vi "Auto_Inspection Station MainS4.vi"(8 "站別":refnum<vi>, 9 "站別":i32, 10 "ActRef":refnum<vi>, 11 "Station Action.lvclass":refnum<class "Station Action.lvclass">) -> ()   [LabVIEW 2019]
uses:
  Station Class/Station Action.lvclass
  Ctrl/Station Action.ctl
  Ctrl/Auto Inspection Data Name.ctl
  FlowCtrl Class/BarcodeScan/Ctl/Board Scan IO.ctl
  FlowCtrl Class/Ctrl/Auto Inspection_IN Name2.ctl
  Ctrl/ModbusCmd.ctl
  Ctrl/S2 Station IO.ctl
  FlowCtrl Class/Laser Detect/Ctl/S11 Station IO.ctl
  Function/Main UI/Glb/Main_UI Gb.vi
  Global/Process Global.vi
  Ctrl/Auto Inspection Main UI Ref.ctl
  LLB/Commonly VI.lvlib
  Ctrl/Auto Inspection Station Name2.ctl
  LLB/Commonly VI/Main Glb.vi
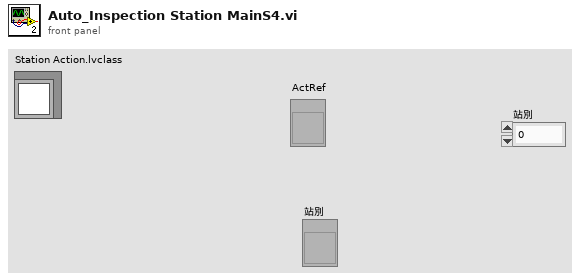
[diagram p1: front panel]
types:
  T1 = typedef "Station Action.ctl" = enum16{"Wait Item In", "Dectect Action", "ImformOut"}
  T2 = cluster{"AutoRunFlg":refnum<vi>, "Action Finish Flg":refnum<vi>, "Remaining Action":refnum<vi>, "Btn_AutoRun":refnum<vi>, "Manual Flg":refnum<vi>, "Sub Process Error":refnum<vi>}
  T3 = typedef "Auto Inspection Data Name.ctl" = enum16{"LocalRun", "ItemSN(TimeCode)", "CurrentAction", "Error", "Data", "OKNG", "電壓值", "電壓值判斷", "電流值", "電流值判斷", "Laser1 Data", "Laser2 Data", "Laser OKNG", "StationNO"}
  T4 = cluster{"starting address":u16, "number of inputs":u16, "Sat Coils":bool[], "Holding Registers":u16[]}
  T5 = typedef "ModbusCmd.ctl" = enum16{"Connect", "Disconnect", "Init", "Fetch Basic Objects", "Fetch Input Refisters", "Fetch Discrete Inputs", "Set Coils", "Set Holding Registers", "Write Single Holding", "Exit"}
  T6 = typedef "Auto Inspection_IN Name2.ctl" = enum16{"S0 Station", "S1 Barcode ", "S2 Tool Format", "S3 Tool Prpgram", "S4 Tool Sacn", "S11 Laser Detect", "S8 Vision AI"}
  T7 = typedef "Board Scan IO.ctl" = enum16{"S1 Barcode Scan", "回給PLC完成讀取訊號", "S1 載盤條碼比對NG", "S1PLC 條碼可讀取訊號", "S1備用_04", "S1備用_05", "S1備用_06", "S1備用_07", "S1備用_08", "S1 發送條碼完成"}
  T8 = typedef "S2 Station IO.ctl" = enum16{"S2站PC動作中_20", "電流量測完成產品OK_21", "電流量測完成產品NG_22", "S2站Format 執行_23", "S2 Format OK_24", "S2 Format NG_25", "S2站燒入執行_26", "S2站燒入OK_27", "S2站燒入NG_28", "S2站動作完成_29", "S3 PC動作中_30", "S3 Format 此站執行_31", "S3 Format OK_32", "S3 Format NG_33", "S3 燒入程式 此站執行_34", "S3 燒入程式 OK_35", "S3 燒入程式 NG_36", "S3 備用_37", "S3 備用_38", "S3 動作完成_39", "S4 PC動作中_40", "S4 量測完成 產品正常_41", "S4 量測完成 產品NG_42", "S4 Format 此站執行_43", "S4 Format OK_44", "S4 Format NG_45", "S4 燒入 此站不執行_46", "S4 燒入程式 OK_47", "S4 燒入程式 NG_48", "S4 藍芽Scan OK_49", "S4 藍芽Scan NG_50", "S4 動作完成_51", "給PLC要量電流訊號", "給PLC要量電壓訊號"}
  T9 = typedef "S11 Station IO.ctl" = enum16{"S11雷射測量動作中", "S11雷射測點1完成", "S11雷射測點2完成", "S11雷測測量OK", "S11雷測測量NG", "S11雷測測量重測", "S11備用_6", "S11備用_7", "S11備用_8", "S11雷射測高完成"}
  T10 = typedef "Auto Inspection Station Name2.ctl" = enum16{"S1Barcode", "S2Measure", "S3Measure", "S4Measure", "S5Measure", "S11_LaserCheck", "S8_Vision AI"}
  T11 = typedef "Auto Inspection Main UI Ref.ctl" = cluster{"LineScan arrive":refnum<vi>, "LineScanfinish":refnum<vi>, "AI arrive":refnum<vi>, "AI finish":refnum<vi>, "NG Pick arrive":refnum<vi>, "NG Pick finish":refnum<vi>}
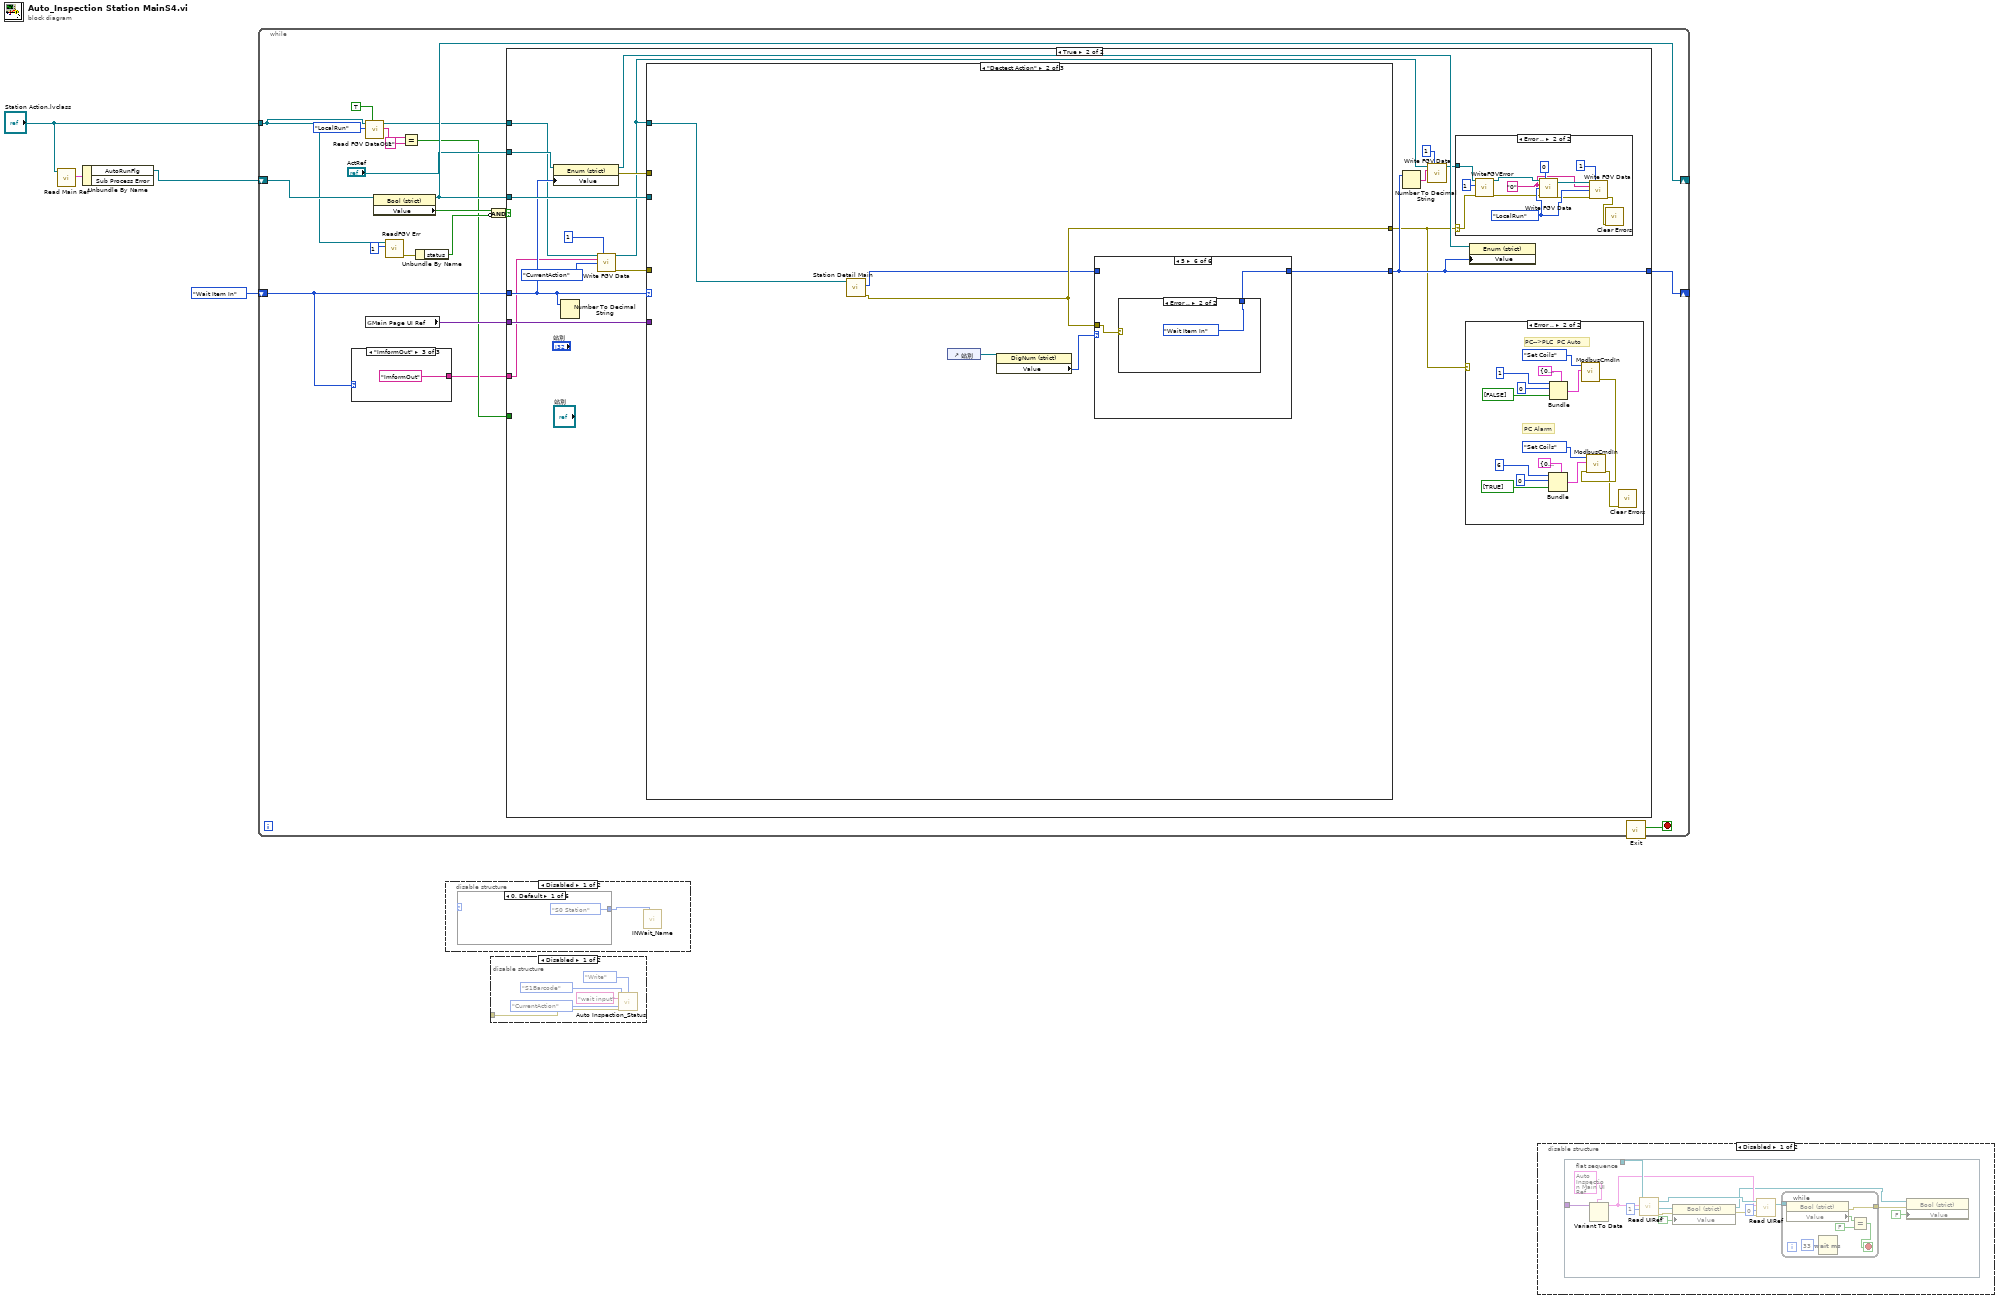
[diagram p0: block diagram]
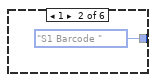
[diagram p2: hidden frame]
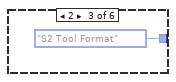
[diagram p3: hidden frame]
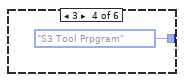
[diagram p4: hidden frame]
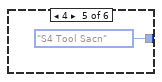
[diagram p5: hidden frame]
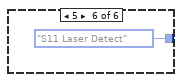
[diagram p6: hidden frame]
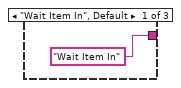
[diagram p10: hidden frame]
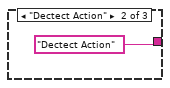
[diagram p11: hidden frame]
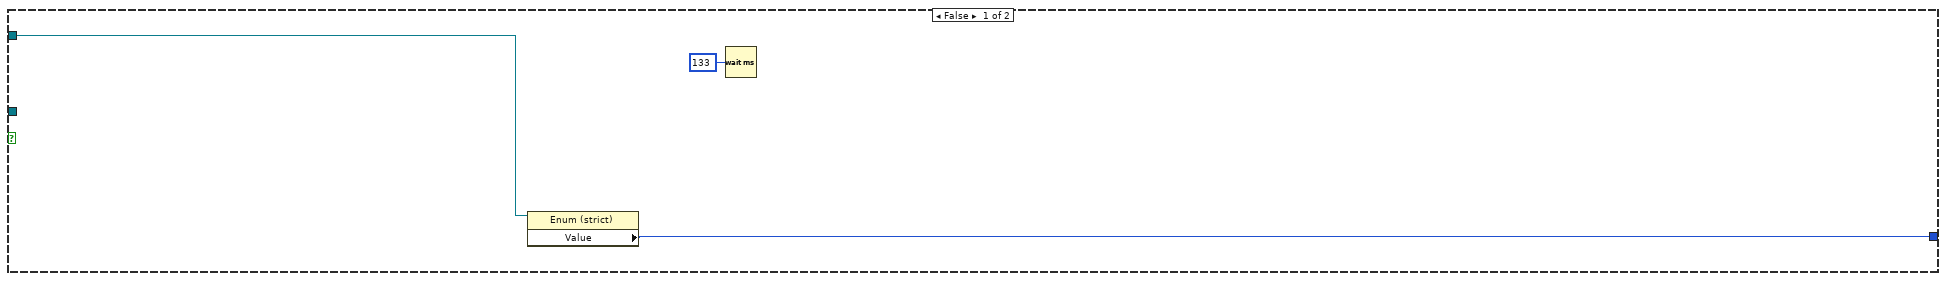
[diagram p12: hidden frame]
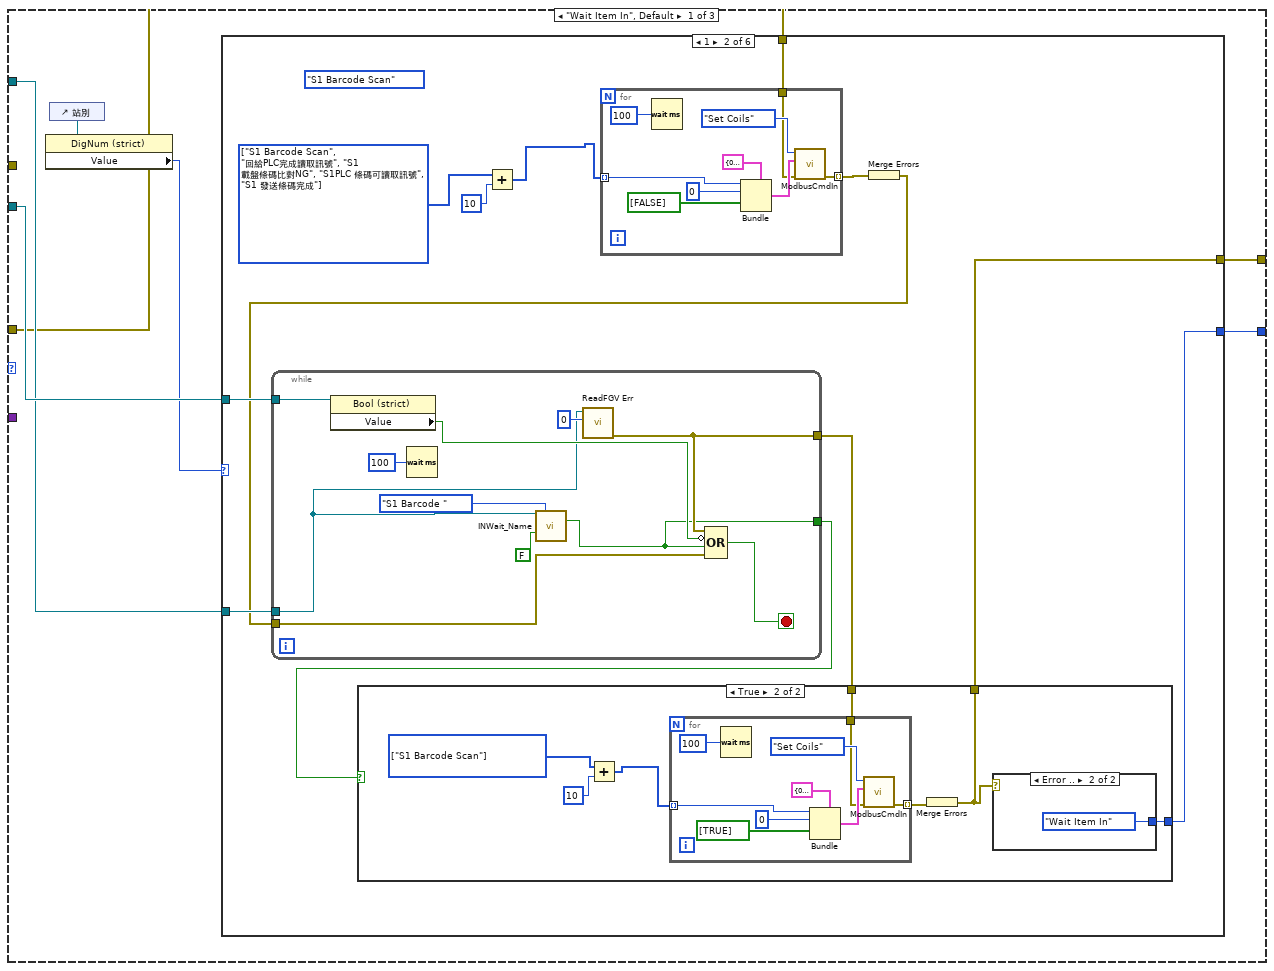
[diagram p15: hidden frame]
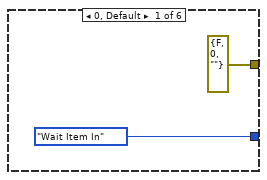
[diagram p16: hidden frame]
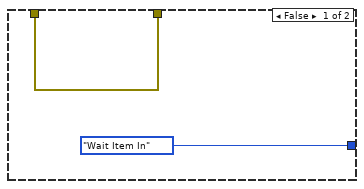
[diagram p17: hidden frame]
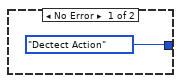
[diagram p18: hidden frame]
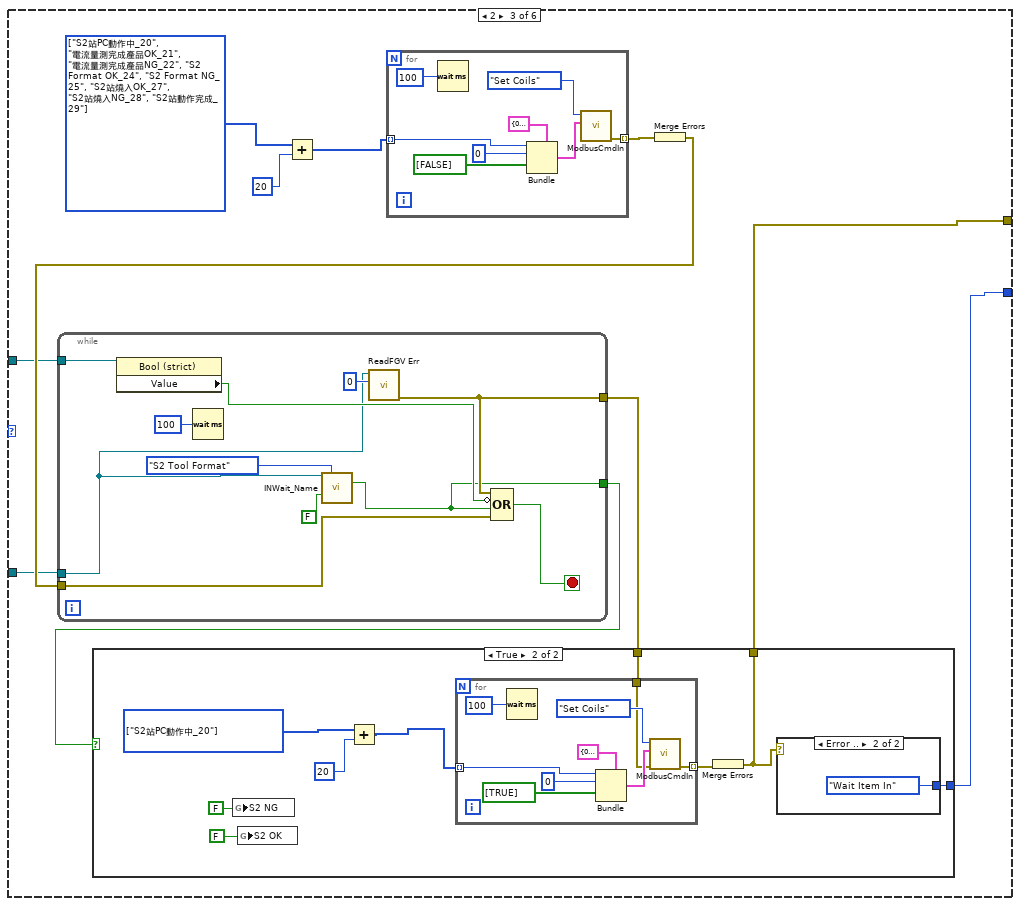
[diagram p19: hidden frame]
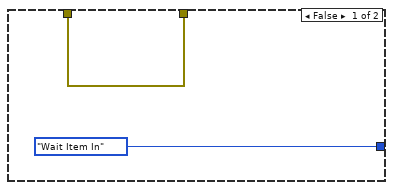
[diagram p20: hidden frame]
diagram:
  n1 = call-dynamic "Read Main Ref.vi"("Main Process Class in"="Station Action.lvclass") -> ("Main Ref"=w3:T2)  [unwired: 8 in, 2 out]
  n2 = Unbundle By Name(w3) -> ("AutoRunFlg"=w1:refnum<vi>)  [unwired: 1 out]
  n3 = while {
    shift-right: [w20] -> _
    shift-left: Station_Action."Wait Item In" -> [w6]
    tunnel: "Station Action.lvclass" -> [w8]
    shift-right: [w18] -> _
    shift-left: w1 -> [w23]
    stop <- w19 stop-if-true
    n4 = case shown="\"ImformOut\"" w6 {
      tunnel: ["Wait Item In" "Dectect Action" "ImformOut"] -> w5
      frame "Wait Item In", Default {
      }
      frame "Dectect Action" {
      }
      frame "ImformOut" {
      }
    }
    n5 = call-dynamic "Read FGV DataOut.vi"("TSt/FConveyor"=TRUE, "Data"=Auto_Inspection_Data_Name."LocalRun", "Station Action in"=w8) -> ("DataOut"=w11:string, "Station Action out"=w14:refnum<class "Station Action.lvclass">)  [unwired: 6 in, 1 out]
    n6 = global read "Main_UI Gb.vi" "Main Page UI Ref"() -> (w21:variant)
    n7 = property class="Bool (strict)"(reference=w23) -> (reference out=w18:refnum<vi>, "Value"=w24:bool)  [unwired: 1 in, 1 out]
    n8 = call-dynamic "ReadFGV Err.vi"("0Cv/1ST"=1, "Station Action in"=w8) -> ("error out"=w16:errorcluster)  [unwired: 8 in, 1 out]
    n9 = Equal?(x=w11, y="1") -> (x = y?=w7:bool)
    n10 = Unbundle By Name(w16) -> ("status"=w15:bool)
    n11 = Compound Arithmetic op=AND(w24, invert w15) -> (w22:bool)
    n12 = case shown="True" w22 {
      tunnel: w18 -> [_ w46]
      tunnel: w6 -> [_ w39]
      tunnel: w21 -> [_ w47]
      tunnel: w14 -> [_ w32]
      tunnel: [w29 w36] -> w20
      tunnel: "ActRef" -> [w30 w45]
      tunnel: w7 -> [_ _]
      tunnel: w5 -> [_ w31]
      frame False {
        n13 = property class="Enum (strict)"(reference=w30) -> ("Value"=w29:T1)  [unwired: 1 in, 2 out]
        n14 = Wait (ms)(milliseconds to wait=u32 133) -> ()  [unwired: 1 out]
      }
      frame True {
        n15 = property class="Enum (strict)"(reference=w45, "Value"=w39) -> (reference out=w44:refnum<vi>, error out=w43:errorcluster)  [unwired: 1 in]
        n16 = Number To Decimal String(number=w39) -> ()  [unwired: 1 in, 1 out]
        n17 = call-dynamic "Write FGV Data.vi"("Station Action in"=w32, "0Cv/1St"=1, "DataIn"=w31, "Data"=Auto_Inspection_Data_Name."CurrentAction") -> ("Station Action out"=w35:refnum<class "Station Action.lvclass">, "error out"=w40:errorcluster)  [unwired: 10 in]
        n18 = case shown="\"Dectect Action\"" w39 {
          tunnel: w47 -> [_ _ _]
          tunnel: w35 -> [w79 w350 w378]
          tunnel: w46 -> [w80 _ w377]
          tunnel: [w75 w348 w373] -> w36
          tunnel: w43 -> [_ _ _]
          tunnel: [w78 w349 w374] -> w33
          tunnel: w40 -> [w74 _ w376]
          frame "Wait Item In", Default {
            n19 = control-ref of="站別"() -> (w77:refnum<vi>)
            n20 = property class="DigNum (strict)"(reference=w77) -> ("Value"=w76:i32)  [unwired: 1 in, 2 out]
            n21 = case shown="1" w76 {
              tunnel: w80 -> [_ w94 w139 w193 w245 w296]
              tunnel: w79 -> [_ w93 w140 w192 w244 w298]
              tunnel: [errorcluster {"status"=FALSE, "code"=0, "source"=""} ("error IO") w92 w142 w195 w241 w297] -> w78
              tunnel: w74 -> [_ w91 _ w188 w246 w299]
              tunnel: [Station_Action."Wait Item In" w87 w141 w194 w243 w294] -> w75
              frame 0, Default {
              }
              frame 1 {
                (unwired) Board_Scan_IO."S1 Barcode Scan" ("Enum")
                w85 = T7[] [enum."S1 Barcode Scan", enum."回給PLC完成讀取訊號", enum."S1 載盤條碼比對NG", enum."S1PLC 條碼可讀取訊號", enum."S1 發送條碼完成"] items=["S1 Barcode Scan", "回給PLC完成讀取訊號", "S1 載盤條碼比對NG", "S1PLC 條碼可讀取訊號", "S1備用_04", "S1備用_05", "S1備用_06", "S1備用_07", "S1備用_08", "S1 發送條碼完成"]
                n22 = Add(x=w85, y=10) -> (x+y=w84:i32[])
                n23 = for {
                  tunnel: [w128] -> w90 mode=indexing
                  tunnel: w84 -> [w127] mode=indexing
                  tunnel: w91 -> [w126]
                  n24 = Wait (ms)(milliseconds to wait=100) -> ()  [unwired: 1 out]
                  n25 = Bundle(cluster=T4 {"starting address"=0, "number of inputs"=0, "Sat Coils"=[], "Holding Registers"=[]} ("data"), "starting address"=w127, "number of inputs"=u16 0, "Sat Coils"=bool[] [FALSE]) -> (w131:T4)  [unwired: 1 in]
                  n26 = call "ModbusCmdIn.vi"("error in (no error)"=w126, "data"=w131, "Enum"=ModbusCmd."Set Coils") -> ("error out"=w128:errorcluster)  [unwired: 8 in]
                }
                n27 = Merge Errors(w90) -> (w89:errorcluster)
                n28 = while {
                  tunnel: w94 -> [w125]
                  tunnel: w93 -> [w119]
                  tunnel: [w120] -> w88
                  tunnel: w89 -> [w117]
                  tunnel: [w116] -> w83
                  stop <- w124 stop-if-true
                  n29 = property class="Bool (strict)"(reference=w125) -> ("Value"=w122:bool)  [unwired: 1 in, 2 out]
                  n30 = Wait (ms)(milliseconds to wait=u32 100) -> ()  [unwired: 1 out]
                  n31 = call "INWait_Name.vi"("FlowCtrl in"=w119, "Input2"=Auto_Inspection_IN_Name2."S1 Barcode ", "Wait?"=FALSE) -> ("StatusOut"=w116:bool)  [unwired: 9 in, 3 out]
                  n32 = call-dynamic "ReadFGV Err.vi"("0Cv/1ST"=0, "Station Action in"=w119) -> ("error out"=w120:errorcluster)  [unwired: 8 in, 1 out]
                  n33 = Compound Arithmetic op=OR(w120, invert w122, w116, w117) -> (w124:bool)
                }
                n34 = case shown="True" w83 {
                  tunnel: [w96 w97] -> w92
                  tunnel: w88 -> [w96 w103]
                  tunnel: [Station_Action."Wait Item In" w100] -> w87
                  frame False {
                  }
                  frame True {
                    w99 = T7[] [enum."S1 Barcode Scan"] items=["S1 Barcode Scan", "回給PLC完成讀取訊號", "S1 載盤條碼比對NG", "S1PLC 條碼可讀取訊號", "S1備用_04", "S1備用_05", "S1備用_06", "S1備用_07", "S1備用_08", "S1 發送條碼完成"]
                    n35 = Add(x=w99, y=10) -> (x+y=w102:i32[])
                    n36 = for {
                      tunnel: [w108] -> w101 mode=indexing
                      tunnel: w102 -> [w107] mode=indexing
                      tunnel: w103 -> [w106]
                      n37 = Wait (ms)(milliseconds to wait=100) -> ()  [unwired: 1 out]
                      n38 = Bundle(cluster=T4 {"starting address"=0, "number of inputs"=0, "Sat Coils"=[], "Holding Registers"=[]} ("data"), "starting address"=w107, "number of inputs"=u16 0, "Sat Coils"=bool[] [TRUE]) -> (w111:T4)  [unwired: 1 in]
                      n39 = call "ModbusCmdIn.vi"("error in (no error)"=w106, "data"=w111, "Enum"=ModbusCmd."Set Coils") -> ("error out"=w108:errorcluster)  [unwired: 8 in]
                    }
                    n40 = Merge Errors(w101) -> (w97:errorcluster)
                    n41 = case shown="Error .." w97 {
                      tunnel: [Station_Action."Dectect Action" Station_Action."Wait Item In"] -> w100
                      frame No Error {
                      }
                      frame Error {
                      }
                    }
                  }
                }
              }
              frame 2 {
                w137 = T8[] [enum."S2站PC動作中_20", enum."電流量測完成產品OK_21", enum."電流量測完成產品NG_22", enum."S2 Format OK_24", enum."S2 Format NG_25", enum."S2站燒入OK_27", enum."S2站燒入NG_28", enum."S2站動作完成_29"] items=["S2站PC動作中_20", "電流量測完成產品OK_21", "電流量測完成產品NG_22", "S2站Format 執行_23", "S2 Format OK_24", "S2 Format NG_25", "S2站燒入執行_26", "S2站燒入OK_27", "S2站燒入NG_28", "S2站動作完成_29", "S3 PC動作中_30", "S3 Format 此站執行_31", "S3 Format OK_32", "S3 Format NG_33", "S3 燒入程式 此站執行_34", "S3 燒入程式 OK_35", "S3 燒入程式 NG_36", "S3 備用_37", "S3 備用_38", "S3 動作完成_39", "S4 PC動作中_40", "S4 量測完成 產品正常_41", "S4 量測完成 產品NG_42", "S4 Format 此站執行_43", "S4 Format OK_44", "S4 Format NG_45", "S4 燒入 此站不執行_46", "S4 燒入程式 OK_47", "S4 燒入程式 NG_48", "S4 藍芽Scan OK_49", "S4 藍芽Scan NG_50", "S4 動作完成_51", "給PLC要量電流訊號", "給PLC要量電壓訊號"]
                n42 = Add(x=w137, y=20) -> (x+y=w136:i32[])
                n43 = for {
                  tunnel: [w180] -> w143 mode=indexing
                  tunnel: w136 -> [w179] mode=indexing
                  n44 = Wait (ms)(milliseconds to wait=100) -> ()  [unwired: 1 out]
                  n45 = Bundle(cluster=T4 {"starting address"=0, "number of inputs"=0, "Sat Coils"=[], "Holding Registers"=[]} ("data"), "starting address"=w179, "number of inputs"=u16 0, "Sat Coils"=bool[] [FALSE]) -> (w183:T4)  [unwired: 1 in]
                  n46 = call "ModbusCmdIn.vi"("data"=w183, "Enum"=ModbusCmd."Set Coils") -> ("error out"=w180:errorcluster)  [unwired: 9 in]
                }
                n47 = Merge Errors(w143) -> (w144:errorcluster)
                n48 = while {
                  tunnel: w140 -> [w173]
                  tunnel: [w174] -> w145
                  tunnel: w144 -> [w171]
                  tunnel: [w170] -> w135
                  tunnel: w139 -> [w168]
                  stop <- w178 stop-if-true
                  n49 = property class="Bool (strict)"(reference=w168) -> ("Value"=w176:bool)  [unwired: 1 in, 2 out]
                  n50 = Wait (ms)(milliseconds to wait=u32 100) -> ()  [unwired: 1 out]
                  n51 = call "INWait_Name.vi"("FlowCtrl in"=w173, "Input2"=Auto_Inspection_IN_Name2."S2 Tool Format", "Wait?"=FALSE) -> ("StatusOut"=w170:bool)  [unwired: 9 in, 3 out]
                  n52 = call-dynamic "ReadFGV Err.vi"("0Cv/1ST"=0, "Station Action in"=w173) -> ("error out"=w174:errorcluster)  [unwired: 8 in, 1 out]
                  n53 = Compound Arithmetic op=OR(w174, invert w176, w170, w171) -> (w178:bool)
                }
                n54 = case shown="True" w135 {
                  tunnel: w145 -> [w147 w155]
                  tunnel: [w147 w150] -> w142
                  tunnel: [Station_Action."Wait Item In" w154] -> w141
                  frame False {
                  }
                  frame True {
                    w153 = T8[] [enum."S2站PC動作中_20"] items=["S2站PC動作中_20", "電流量測完成產品OK_21", "電流量測完成產品NG_22", "S2站Format 執行_23", "S2 Format OK_24", "S2 Format NG_25", "S2站燒入執行_26", "S2站燒入OK_27", "S2站燒入NG_28", "S2站動作完成_29", "S3 PC動作中_30", "S3 Format 此站執行_31", "S3 Format OK_32", "S3 Format NG_33", "S3 燒入程式 此站執行_34", "S3 燒入程式 OK_35", "S3 燒入程式 NG_36", "S3 備用_37", "S3 備用_38", "S3 動作完成_39", "S4 PC動作中_40", "S4 量測完成 產品正常_41", "S4 量測完成 產品NG_42", "S4 Format 此站執行_43", "S4 Format OK_44", "S4 Format NG_45", "S4 燒入 此站不執行_46", "S4 燒入程式 OK_47", "S4 燒入程式 NG_48", "S4 藍芽Scan OK_49", "S4 藍芽Scan NG_50", "S4 動作完成_51", "給PLC要量電流訊號", "給PLC要量電壓訊號"]
                    n55 = global write "Process Global.vi" "S2 NG"(FALSE) -> ()
                    n56 = global write "Process Global.vi" "S2 OK"(FALSE) -> ()
                    n57 = Add(x=w153, y=20) -> (x+y=w151:i32[])
                    n58 = for {
                      tunnel: [w161] -> w156 mode=indexing
                      tunnel: w151 -> [w160] mode=indexing
                      tunnel: w155 -> [w159]
                      n59 = Wait (ms)(milliseconds to wait=100) -> ()  [unwired: 1 out]
                      n60 = Bundle(cluster=T4 {"starting address"=0, "number of inputs"=0, "Sat Coils"=[], "Holding Registers"=[]} ("data"), "starting address"=w160, "number of inputs"=u16 0, "Sat Coils"=bool[] [TRUE]) -> (w164:T4)  [unwired: 1 in]
                      n61 = call "ModbusCmdIn.vi"("error in (no error)"=w159, "data"=w164, "Enum"=ModbusCmd."Set Coils") -> ("error out"=w161:errorcluster)  [unwired: 8 in]
                    }
                    n62 = Merge Errors(w156) -> (w150:errorcluster)
                    n63 = case shown="Error .." w150 {
                      tunnel: [Station_Action."Dectect Action" Station_Action."Wait Item In"] -> w154
                      frame No Error {
                      }
                      frame Error {
                      }
                    }
                  }
                }
              }
              frame 3 {
                w191 = T8[] [enum."S3 PC動作中_30", enum."S3 Format OK_32", enum."S3 Format NG_33", enum."S3 燒入程式 OK_35", enum."S3 燒入程式 NG_36", enum."S3 動作完成_39"] items=["S2站PC動作中_20", "電流量測完成產品OK_21", "電流量測完成產品NG_22", "S2站Format 執行_23", "S2 Format OK_24", "S2 Format NG_25", "S2站燒入執行_26", "S2站燒入OK_27", "S2站燒入NG_28", "S2站動作完成_29", "S3 PC動作中_30", "S3 Format 此站執行_31", "S3 Format OK_32", "S3 Format NG_33", "S3 燒入程式 此站執行_34", "S3 燒入程式 OK_35", "S3 燒入程式 NG_36", "S3 備用_37", "S3 備用_38", "S3 動作完成_39", "S4 PC動作中_40", "S4 量測完成 產品正常_41", "S4 量測完成 產品NG_42", "S4 Format 此站執行_43", "S4 Format OK_44", "S4 Format NG_45", "S4 燒入 此站不執行_46", "S4 燒入程式 OK_47", "S4 燒入程式 NG_48", "S4 藍芽Scan OK_49", "S4 藍芽Scan NG_50", "S4 動作完成_51", "給PLC要量電流訊號", "給PLC要量電壓訊號"]
                n64 = Add(x=w191, y=20) -> (x+y=w189:i32[])
                n65 = for {
                  tunnel: [w233] -> w196 mode=indexing
                  tunnel: w189 -> [w232] mode=indexing
                  tunnel: w188 -> [w231]
                  n66 = Wait (ms)(milliseconds to wait=100) -> ()  [unwired: 1 out]
                  n67 = Bundle(cluster=T4 {"starting address"=0, "number of inputs"=0, "Sat Coils"=[], "Holding Registers"=[]} ("data"), "starting address"=w232, "number of inputs"=u16 0, "Sat Coils"=bool[] [FALSE]) -> (w236:T4)  [unwired: 1 in]
                  n68 = call "ModbusCmdIn.vi"("error in (no error)"=w231, "data"=w236, "Enum"=ModbusCmd."Set Coils") -> ("error out"=w233:errorcluster)  [unwired: 8 in]
                }
                n69 = Merge Errors(w196) -> (w197:errorcluster)
                n70 = while {
                  tunnel: w193 -> [w230]
                  tunnel: w192 -> [w224]
                  tunnel: [w225] -> w198
                  tunnel: w197 -> [w222]
                  tunnel: [w221] -> w187
                  stop <- w229 stop-if-true
                  n71 = property class="Bool (strict)"(reference=w230) -> ("Value"=w227:bool)  [unwired: 1 in, 2 out]
                  n72 = Wait (ms)(milliseconds to wait=u32 100) -> ()  [unwired: 1 out]
                  n73 = call "INWait_Name.vi"("FlowCtrl in"=w224, "Input2"=Auto_Inspection_IN_Name2."S3 Tool Prpgram", "Wait?"=FALSE) -> ("StatusOut"=w221:bool)  [unwired: 9 in, 3 out]
                  n74 = call-dynamic "ReadFGV Err.vi"("0Cv/1ST"=0, "Station Action in"=w224) -> ("error out"=w225:errorcluster)  [unwired: 8 in, 1 out]
                  n75 = Compound Arithmetic op=OR(w225, invert w227, w221, w222) -> (w229:bool)
                }
                n76 = case shown="True" w187 {
                  tunnel: w198 -> [w200 w207]
                  tunnel: [w200 w202] -> w195
                  tunnel: [Station_Action."Wait Item In" w206] -> w194
                  frame False {
                  }
                  frame True {
                    w201 = FALSE ("S3 NG")
                    w204 = T8[] [enum."S3 PC動作中_30"] items=["S2站PC動作中_20", "電流量測完成產品OK_21", "電流量測完成產品NG_22", "S2站Format 執行_23", "S2 Format OK_24", "S2 Format NG_25", "S2站燒入執行_26", "S2站燒入OK_27", "S2站燒入NG_28", "S2站動作完成_29", "S3 PC動作中_30", "S3 Format 此站執行_31", "S3 Format OK_32", "S3 Format NG_33", "S3 燒入程式 此站執行_34", "S3 燒入程式 OK_35", "S3 燒入程式 NG_36", "S3 備用_37", "S3 備用_38", "S3 動作完成_39", "S4 PC動作中_40", "S4 量測完成 產品正常_41", "S4 量測完成 產品NG_42", "S4 Format 此站執行_43", "S4 Format OK_44", "S4 Format NG_45", "S4 燒入 此站不執行_46", "S4 燒入程式 OK_47", "S4 燒入程式 NG_48", "S4 藍芽Scan OK_49", "S4 藍芽Scan NG_50", "S4 動作完成_51", "給PLC要量電流訊號", "給PLC要量電壓訊號"]
                    n77 = global write "Process Global.vi" "S3 NG"(w201) -> ()
                    n78 = global write "Process Global.vi" "S3 OK"(w201) -> ()
                    n79 = Add(x=w204, y=20) -> (x+y=w203:i32[])
                    n80 = for {
                      tunnel: [w213] -> w208 mode=indexing
                      tunnel: w203 -> [w212] mode=indexing
                      tunnel: w207 -> [w211]
                      n81 = Wait (ms)(milliseconds to wait=100) -> ()  [unwired: 1 out]
                      n82 = Bundle(cluster=T4 {"starting address"=0, "number of inputs"=0, "Sat Coils"=[], "Holding Registers"=[]} ("data"), "starting address"=w212, "number of inputs"=u16 0, "Sat Coils"=bool[] [TRUE]) -> (w216:T4)  [unwired: 1 in]
                      n83 = call "ModbusCmdIn.vi"("error in (no error)"=w211, "data"=w216, "Enum"=ModbusCmd."Set Coils") -> ("error out"=w213:errorcluster)  [unwired: 8 in]
                    }
                    n84 = Merge Errors(w208) -> (w202:errorcluster)
                    n85 = case shown="Error .." w202 {
                      tunnel: [Station_Action."Dectect Action" Station_Action."Wait Item In"] -> w206
                      frame No Error {
                      }
                      frame Error {
                      }
                    }
                  }
                }
              }
              frame 4 {
                w242 = T8[] [enum."S4 PC動作中_40", enum."S4 量測完成 產品正常_41", enum."S4 量測完成 產品NG_42", enum."S4 Format OK_44", enum."S4 Format NG_45", enum."S4 燒入程式 OK_47", enum."S4 燒入程式 NG_48", enum."S4 藍芽Scan OK_49", enum."S4 藍芽Scan NG_50", enum."S4 動作完成_51"] items=["S2站PC動作中_20", "電流量測完成產品OK_21", "電流量測完成產品NG_22", "S2站Format 執行_23", "S2 Format OK_24", "S2 Format NG_25", "S2站燒入執行_26", "S2站燒入OK_27", "S2站燒入NG_28", "S2站動作完成_29", "S3 PC動作中_30", "S3 Format 此站執行_31", "S3 Format OK_32", "S3 Format NG_33", "S3 燒入程式 此站執行_34", "S3 燒入程式 OK_35", "S3 燒入程式 NG_36", "S3 備用_37", "S3 備用_38", "S3 動作完成_39", "S4 PC動作中_40", "S4 量測完成 產品正常_41", "S4 量測完成 產品NG_42", "S4 Format 此站執行_43", "S4 Format OK_44", "S4 Format NG_45", "S4 燒入 此站不執行_46", "S4 燒入程式 OK_47", "S4 燒入程式 NG_48", "S4 藍芽Scan OK_49", "S4 藍芽Scan NG_50", "S4 動作完成_51", "給PLC要量電流訊號", "給PLC要量電壓訊號"]
                n86 = Add(x=w242, y=20) -> (x+y=w251:i32[])
                n87 = for {
                  tunnel: [w286] -> w247 mode=indexing
                  tunnel: w251 -> [w285] mode=indexing
                  tunnel: w246 -> [w284]
                  n88 = Wait (ms)(milliseconds to wait=100) -> ()  [unwired: 1 out]
                  n89 = Bundle(cluster=T4 {"starting address"=0, "number of inputs"=0, "Sat Coils"=[], "Holding Registers"=[]} ("data"), "starting address"=w285, "number of inputs"=u16 0, "Sat Coils"=bool[] [FALSE]) -> (w289:T4)  [unwired: 1 in]
                  n90 = call "ModbusCmdIn.vi"("error in (no error)"=w284, "data"=w289, "Enum"=ModbusCmd."Set Coils") -> ("error out"=w286:errorcluster)  [unwired: 8 in]
                }
                n91 = Merge Errors(w247) -> (w248:errorcluster)
                n92 = while {
                  tunnel: [w279] -> w249
                  tunnel: w248 -> [w277]
                  tunnel: [w276] -> w240
                  tunnel: w245 -> [w274]
                  tunnel: w244 -> [w273]
                  stop <- w283 stop-if-true
                  n93 = property class="Bool (strict)"(reference=w274) -> ("Value"=w281:bool)  [unwired: 1 in, 2 out]
                  n94 = Wait (ms)(milliseconds to wait=u32 100) -> ()  [unwired: 1 out]
                  n95 = call "INWait_Name.vi"("FlowCtrl in"=w273, "Input2"=Auto_Inspection_IN_Name2."S4 Tool Sacn", "Wait?"=FALSE) -> ("StatusOut"=w276:bool)  [unwired: 9 in, 3 out]
                  n96 = call-dynamic "ReadFGV Err.vi"("0Cv/1ST"=0, "Station Action in"=w273) -> ("error out"=w279:errorcluster)  [unwired: 8 in, 1 out]
                  n97 = Compound Arithmetic op=OR(w279, invert w281, w276, w277) -> (w283:bool)
                }
                n98 = case shown="True" w240 {
                  tunnel: w249 -> [w253 w258]
                  tunnel: [Station_Action."Wait Item In" w257] -> w243
                  tunnel: [w253 w255] -> w241
                  frame False {
                  }
                  frame True {
                    w254 = FALSE ("S4 NG")
                    w256 = T8[] [enum."S4 PC動作中_40"] items=["S2站PC動作中_20", "電流量測完成產品OK_21", "電流量測完成產品NG_22", "S2站Format 執行_23", "S2 Format OK_24", "S2 Format NG_25", "S2站燒入執行_26", "S2站燒入OK_27", "S2站燒入NG_28", "S2站動作完成_29", "S3 PC動作中_30", "S3 Format 此站執行_31", "S3 Format OK_32", "S3 Format NG_33", "S3 燒入程式 此站執行_34", "S3 燒入程式 OK_35", "S3 燒入程式 NG_36", "S3 備用_37", "S3 備用_38", "S3 動作完成_39", "S4 PC動作中_40", "S4 量測完成 產品正常_41", "S4 量測完成 產品NG_42", "S4 Format 此站執行_43", "S4 Format OK_44", "S4 Format NG_45", "S4 燒入 此站不執行_46", "S4 燒入程式 OK_47", "S4 燒入程式 NG_48", "S4 藍芽Scan OK_49", "S4 藍芽Scan NG_50", "S4 動作完成_51", "給PLC要量電流訊號", "給PLC要量電壓訊號"]
                    n99 = global write "Process Global.vi" "S4 NG"(w254) -> ()
                    n100 = global write "Process Global.vi" "S4 OK"(w254) -> ()
                    n101 = Add(x=w256, y=20) -> (x+y=w259:i32[])
                    n102 = for {
                      tunnel: [w266] -> w260 mode=indexing
                      tunnel: w259 -> [w265] mode=indexing
                      tunnel: w258 -> [w264]
                      n103 = Wait (ms)(milliseconds to wait=100) -> ()  [unwired: 1 out]
                      n104 = Bundle(cluster=T4 {"starting address"=0, "number of inputs"=0, "Sat Coils"=[], "Holding Registers"=[]} ("data"), "starting address"=w265, "number of inputs"=u16 0, "Sat Coils"=bool[] [TRUE]) -> (w269:T4)  [unwired: 1 in]
                      n105 = call "ModbusCmdIn.vi"("error in (no error)"=w264, "data"=w269, "Enum"=ModbusCmd."Set Coils") -> ("error out"=w266:errorcluster)  [unwired: 8 in]
                    }
                    n106 = Merge Errors(w260) -> (w255:errorcluster)
                    n107 = case shown="Error .." w255 {
                      tunnel: [Station_Action."Dectect Action" Station_Action."Wait Item In"] -> w257
                      frame No Error {
                      }
                      frame Error {
                      }
                    }
                  }
                }
              }
              frame 5 {
                w295 = T9[] [enum."S11雷射測量動作中", enum."S11雷測測量OK", enum."S11雷測測量OK", enum."S11雷測測量NG", enum."S11雷測測量重測", enum."S11雷射測高完成"] items=["S11雷射測量動作中", "S11雷射測點1完成", "S11雷射測點2完成", "S11雷測測量OK", "S11雷測測量NG", "S11雷測測量重測", "S11備用_6", "S11備用_7", "S11備用_8", "S11雷射測高完成"]
                n108 = Add(x=w295, y=110) -> (x+y=w304:i32[])
                n109 = for {
                  tunnel: [w338] -> w300 mode=indexing
                  tunnel: w304 -> [w337] mode=indexing
                  tunnel: w299 -> [w336]
                  n110 = Wait (ms)(milliseconds to wait=100) -> ()  [unwired: 1 out]
                  n111 = Bundle(cluster=T4 {"starting address"=0, "number of inputs"=0, "Sat Coils"=[], "Holding Registers"=[]} ("data"), "starting address"=w337, "number of inputs"=u16 0, "Sat Coils"=bool[] [FALSE]) -> (w341:T4)  [unwired: 1 in]
                  n112 = call "ModbusCmdIn.vi"("error in (no error)"=w336, "data"=w341, "Enum"=ModbusCmd."Set Coils") -> ("error out"=w338:errorcluster)  [unwired: 8 in]
                }
                n113 = Merge Errors(w300) -> (w301:errorcluster)
                n114 = while {
                  tunnel: [w331] -> w302
                  tunnel: w301 -> [w329]
                  tunnel: [w328] -> w293
                  tunnel: w298 -> [w325]
                  tunnel: w296 -> [w326]
                  stop <- w335 stop-if-true
                  n115 = property class="Bool (strict)"(reference=w326) -> ("Value"=w333:bool)  [unwired: 1 in, 2 out]
                  n116 = Wait (ms)(milliseconds to wait=u32 100) -> ()  [unwired: 1 out]
                  n117 = call "INWait_Name.vi"("FlowCtrl in"=w325, "Input2"=Auto_Inspection_IN_Name2."S11 Laser Detect", "Wait?"=FALSE) -> ("StatusOut"=w328:bool)  [unwired: 9 in, 3 out]
                  n118 = call-dynamic "ReadFGV Err.vi"("0Cv/1ST"=0, "Station Action in"=w325) -> ("error out"=w331:errorcluster)  [unwired: 8 in, 1 out]
                  n119 = Compound Arithmetic op=OR(w331, invert w333, w328, w329) -> (w335:bool)
                }
                n120 = case shown="True" w293 {
                  tunnel: w302 -> [w305 w310]
                  tunnel: [w305 w308] -> w297
                  tunnel: [Station_Action."Wait Item In" w307] -> w294
                  frame False {
                  }
                  frame True {
                    w309 = T9[] [enum."S11雷射測量動作中"] items=["S11雷射測量動作中", "S11雷射測點1完成", "S11雷射測點2完成", "S11雷測測量OK", "S11雷測測量NG", "S11雷測測量重測", "S11備用_6", "S11備用_7", "S11備用_8", "S11雷射測高完成"]
                    n121 = Add(x=w309, y=110) -> (x+y=w311:i32[])
                    n122 = for {
                      tunnel: [w318] -> w312 mode=indexing
                      tunnel: w311 -> [w317] mode=indexing
                      tunnel: w310 -> [w316]
                      n123 = Wait (ms)(milliseconds to wait=100) -> ()  [unwired: 1 out]
                      n124 = Bundle(cluster=T4 {"starting address"=0, "number of inputs"=0, "Sat Coils"=[], "Holding Registers"=[]} ("data"), "starting address"=w317, "number of inputs"=u16 0, "Sat Coils"=bool[] [TRUE]) -> (w321:T4)  [unwired: 1 in]
                      n125 = call "ModbusCmdIn.vi"("error in (no error)"=w316, "data"=w321, "Enum"=ModbusCmd."Set Coils") -> ("error out"=w318:errorcluster)  [unwired: 8 in]
                    }
                    n126 = Merge Errors(w312) -> (w308:errorcluster)
                    n127 = case shown="Error .." w308 {
                      tunnel: [Station_Action."Dectect Action" Station_Action."Wait Item In"] -> w307
                      frame No Error {
                      }
                      frame Error {
                      }
                    }
                  }
                }
              }
            }
          }
          frame "Dectect Action" {
            n128 = call-dynamic "Station Detail Main.vi"("Station Action in"=w350) -> ("error out"=w349:errorcluster, "Station Out"=w345:T1)  [unwired: 8 in, 1 out]
            n129 = control-ref of="站別"() -> (w347:refnum<vi>)
            n130 = property class="DigNum (strict)"(reference=w347) -> ("Value"=w346:i32)  [unwired: 1 in, 2 out]
            n131 = case shown="5" w346 {
              tunnel: w349 -> [_ w353 w356 w360 w364 w368]
              tunnel: [w351 w352 w357 w361 w365 w369] -> w348
              tunnel: w345 -> [w351 _ _ _ _ _]
              frame 0, Default {
              }
              frame 1 {
                n132 = case shown="Error .." w353 {
                  tunnel: [Station_Action."ImformOut" ("Station Out") Station_Action."Wait Item In" ("Station Out")] -> w352
                  frame No Error {
                  }
                  frame Error {
                  }
                }
              }
              frame 2 {
                n133 = case shown="Error .." w356 {
                  tunnel: [Station_Action."ImformOut" ("Station Out") Station_Action."Wait Item In" ("Station Out")] -> w357
                  frame No Error {
                  }
                  frame Error {
                  }
                }
              }
              frame 3 {
                n134 = case shown="Error .." w360 {
                  tunnel: [Station_Action."ImformOut" ("Station Out") Station_Action."Wait Item In" ("Station Out")] -> w361
                  frame No Error {
                  }
                  frame Error {
                  }
                }
              }
              frame 4 {
                n135 = case shown="Error .." w364 {
                  tunnel: [Station_Action."ImformOut" ("Station Out") Station_Action."Wait Item In" ("Station Out")] -> w365
                  frame No Error {
                  }
                  frame Error {
                  }
                }
              }
              frame 5 {
                n136 = case shown="Error .." w368 {
                  tunnel: [Station_Action."ImformOut" ("Station Out") Station_Action."Wait Item In" ("Station Out")] -> w369
                  frame No Error {
                  }
                  frame Error {
                  }
                }
              }
            }
          }
          frame "ImformOut" {
            # "AutoRunFlg"
            n137 = control-ref of="站別"() -> (w375:refnum<vi>)
            n138 = property class="DigNum (strict)"(reference=w375) -> ("Value"=w372:i32)  [unwired: 1 in, 2 out]
            n139 = case shown="5" w372 {
              selector: w372 -> [_ _ _ w495 _ _]
              tunnel: w378 -> [_ w393 w440 w497 w553 w623]
              tunnel: w377 -> [_ w392 w439 w496 w552 w622]
              tunnel: w376 -> [_ w391 w443 w500 w554 w624]
              tunnel: w372 -> [_ _ _ _ _ _]
              tunnel: [errorcluster {"status"=FALSE, "code"=0, "source"=""} ("error IO") w384 w438 w493 w556 w620] -> w374
              tunnel: [Station_Action."Wait Item In" w383 w437 w494 w555 w621] -> w373
              frame 0, Default {
              }
              frame 1 {
                w382 = T7[] [enum."S1 Barcode Scan"] items=["S1 Barcode Scan", "回給PLC完成讀取訊號", "S1 載盤條碼比對NG", "S1PLC 條碼可讀取訊號", "S1備用_04", "S1備用_05", "S1備用_06", "S1備用_07", "S1備用_08", "S1 發送條碼完成"]
                n140 = Add(x=w382, y=10) -> (x+y=w390:i32[])
                n141 = for {
                  tunnel: [w399] -> w389 mode=indexing
                  tunnel: w391 -> [w398]
                  tunnel: w390 -> [w397] mode=indexing
                  tunnel: bool[] [FALSE] ("Sat Coils") -> [w396]
                  n142 = Wait (ms)(milliseconds to wait=100) -> ()  [unwired: 1 out]
                  n143 = Bundle(cluster=T4 {"starting address"=0, "number of inputs"=0, "Sat Coils"=[], "Holding Registers"=[]} ("data"), "starting address"=w397, "number of inputs"=u16 0, "Sat Coils"=w396) -> (w402:T4)  [unwired: 1 in]
                  n144 = call "ModbusCmdIn.vi"("error in (no error)"=w398, "data"=w402, "Enum"=ModbusCmd."Set Coils") -> ("error out"=w399:errorcluster)  [unwired: 8 in]
                }
                n145 = Merge Errors(w389) -> (w388:errorcluster)
                n146 = while {
                  tunnel: w393 -> [w435]
                  tunnel: w392 -> [w434]
                  tunnel: [w427] -> w387
                  tunnel: [w430] -> w386
                  tunnel: w388 -> [w424]
                  stop <- w431 stop-if-true
                  n147 = property class="Bool (strict)"(reference=w434) -> ("Value"=w433:bool)  [unwired: 1 in, 2 out]
                  n148 = Not(x=w433) -> (.not. x?=w432:bool)
                  n149 = call "INWait_Name.vi"("FlowCtrl in"=w435, "Input2"=Auto_Inspection_IN_Name2."S1 Barcode ", "Wait?"=FALSE, "error in (no error)"=w424) -> ("StatusOut"=w429:bool, "error out"=w430:errorcluster)  [unwired: 8 in, 2 out]
                  n150 = Equal?(x=FALSE, y=w429) -> (x = y?=w427:bool)
                  n151 = Compound Arithmetic op=OR(w424, w427, w432) -> (w431:bool)
                  n152 = Wait (ms)(milliseconds to wait=123) -> ()  [unwired: 1 out]
                }
                n153 = case shown="True" w387 {
                  tunnel: w386 -> [w405 w411]
                  tunnel: [w405 w408] -> w384
                  frame False {
                  }
                  frame True {
                    w407 = T7[] [enum."S1 Barcode Scan", enum."回給PLC完成讀取訊號", enum."S1 載盤條碼比對NG", enum."S1PLC 條碼可讀取訊號", enum."S1 發送條碼完成"] items=["S1 Barcode Scan", "回給PLC完成讀取訊號", "S1 載盤條碼比對NG", "S1PLC 條碼可讀取訊號", "S1備用_04", "S1備用_05", "S1備用_06", "S1備用_07", "S1備用_08", "S1 發送條碼完成"]
                    n154 = Add(x=w407, y=10) -> (x+y=w410:i32[])
                    n155 = for {
                      tunnel: w410 -> [w415] mode=indexing
                      tunnel: [w417] -> w412 mode=indexing
                      tunnel: w411 -> [w416]
                      n156 = Wait (ms)(milliseconds to wait=100) -> ()  [unwired: 1 out]
                      n157 = Bundle(cluster=T4 {"starting address"=0, "number of inputs"=0, "Sat Coils"=[], "Holding Registers"=[]} ("data"), "starting address"=w415, "number of inputs"=u16 0, "Sat Coils"=bool[] [FALSE]) -> (w420:T4)  [unwired: 1 in]
                      n158 = call "ModbusCmdIn.vi"("error in (no error)"=w416, "data"=w420, "Enum"=ModbusCmd."Set Coils") -> ("error out"=w417:errorcluster)  [unwired: 8 in]
                    }
                    n159 = Merge Errors(w412) -> (w409:errorcluster)
                    n160 = case shown="No Error" w409 {
                      selector: w409 -> [w413 w414]
                      tunnel: [w413 w414] -> w408
                      frame No Error {
                      }
                      frame Error {
                      }
                    }
                  }
                }
                n161 = case shown="No Error" w384 {
                  tunnel: [Station_Action."Wait Item In" Station_Action."ImformOut"] -> w383
                  frame No Error {
                  }
                  frame Error {
                  }
                }
              }
              frame 2 {
                w441 = T8[] [enum."S2站動作完成_29"] items=["S2站PC動作中_20", "電流量測完成產品OK_21", "電流量測完成產品NG_22", "S2站Format 執行_23", "S2 Format OK_24", "S2 Format NG_25", "S2站燒入執行_26", "S2站燒入OK_27", "S2站燒入NG_28", "S2站動作完成_29", "S3 PC動作中_30", "S3 Format 此站執行_31", "S3 Format OK_32", "S3 Format NG_33", "S3 燒入程式 此站執行_34", "S3 燒入程式 OK_35", "S3 燒入程式 NG_36", "S3 備用_37", "S3 備用_38", "S3 動作完成_39", "S4 PC動作中_40", "S4 量測完成 產品正常_41", "S4 量測完成 產品NG_42", "S4 Format 此站執行_43", "S4 Format OK_44", "S4 Format NG_45", "S4 燒入 此站不執行_46", "S4 燒入程式 OK_47", "S4 燒入程式 NG_48", "S4 藍芽Scan OK_49", "S4 藍芽Scan NG_50", "S4 動作完成_51", "給PLC要量電流訊號", "給PLC要量電壓訊號"]
                n162 = Add(x=w441, y=20) -> (x+y=w449:i32[])
                n163 = for {
                  tunnel: [w455] -> w448 mode=indexing
                  tunnel: w443 -> [w454]
                  tunnel: w449 -> [w453] mode=indexing
                  tunnel: bool[] [TRUE] ("Sat Coils") -> [w452]
                  n164 = Wait (ms)(milliseconds to wait=100) -> ()  [unwired: 1 out]
                  n165 = Bundle(cluster=T4 {"starting address"=0, "number of inputs"=0, "Sat Coils"=[], "Holding Registers"=[]} ("data"), "starting address"=w453, "number of inputs"=u16 0, "Sat Coils"=w452) -> (w458:T4)  [unwired: 1 in]
                  n166 = call "ModbusCmdIn.vi"("error in (no error)"=w454, "data"=w458, "Enum"=ModbusCmd."Set Coils") -> ("error out"=w455:errorcluster)  [unwired: 8 in]
                }
                n167 = Merge Errors(w448) -> (w447:errorcluster)
                n168 = while {
                  tunnel: w440 -> [w491]
                  tunnel: w439 -> [w490]
                  tunnel: [w483] -> w446
                  tunnel: [w486] -> w445
                  tunnel: w447 -> [w480]
                  stop <- w487 stop-if-true
                  n169 = property class="Bool (strict)"(reference=w490) -> ("Value"=w489:bool)  [unwired: 1 in, 2 out]
                  n170 = Not(x=w489) -> (.not. x?=w488:bool)
                  n171 = call "INWait_Name.vi"("FlowCtrl in"=w491, "Input2"=Auto_Inspection_IN_Name2."S2 Tool Format", "Wait?"=FALSE, "error in (no error)"=w480) -> ("StatusOut"=w485:bool, "error out"=w486:errorcluster)  [unwired: 8 in, 2 out]
                  n172 = Equal?(x=FALSE, y=w485) -> (x = y?=w483:bool)
                  n173 = Compound Arithmetic op=OR(w480, w483, w488) -> (w487:bool)
                  n174 = Wait (ms)(milliseconds to wait=123) -> ()  [unwired: 1 out]
                }
                n175 = case shown="True" w446 {
                  tunnel: w445 -> [w461 w467]
                  tunnel: [w461 w462] -> w438
                  frame False {
                  }
                  frame True {
                    w463 = T8[] [enum."S2站PC動作中_20", enum."電流量測完成產品OK_21", enum."電流量測完成產品NG_22", enum."S2站Format 執行_23", enum."S2 Format OK_24", enum."S2 Format NG_25", enum."S2站燒入執行_26", enum."S2站燒入OK_27", enum."S2站燒入NG_28", enum."S2站動作完成_29", enum."給PLC要量電流訊號"] items=["S2站PC動作中_20", "電流量測完成產品OK_21", "電流量測完成產品NG_22", "S2站Format 執行_23", "S2 Format OK_24", "S2 Format NG_25", "S2站燒入執行_26", "S2站燒入OK_27", "S2站燒入NG_28", "S2站動作完成_29", "S3 PC動作中_30", "S3 Format 此站執行_31", "S3 Format OK_32", "S3 Format NG_33", "S3 燒入程式 此站執行_34", "S3 燒入程式 OK_35", "S3 燒入程式 NG_36", "S3 備用_37", "S3 備用_38", "S3 動作完成_39", "S4 PC動作中_40", "S4 量測完成 產品正常_41", "S4 量測完成 產品NG_42", "S4 Format 此站執行_43", "S4 Format OK_44", "S4 Format NG_45", "S4 燒入 此站不執行_46", "S4 燒入程式 OK_47", "S4 燒入程式 NG_48", "S4 藍芽Scan OK_49", "S4 藍芽Scan NG_50", "S4 動作完成_51", "給PLC要量電流訊號", "給PLC要量電壓訊號"]
                    n176 = Add(x=w463, y=20) -> (x+y=w466:i32[])
                    n177 = for {
                      tunnel: w466 -> [w471] mode=indexing
                      tunnel: [w473] -> w468 mode=indexing
                      tunnel: w467 -> [w472]
                      n178 = Wait (ms)(milliseconds to wait=100) -> ()  [unwired: 1 out]
                      n179 = Bundle(cluster=T4 {"starting address"=0, "number of inputs"=0, "Sat Coils"=[], "Holding Registers"=[]} ("data"), "starting address"=w471, "number of inputs"=u16 0, "Sat Coils"=bool[] [FALSE]) -> (w476:T4)  [unwired: 1 in]
                      n180 = call "ModbusCmdIn.vi"("error in (no error)"=w472, "data"=w476, "Enum"=ModbusCmd."Set Coils") -> ("error out"=w473:errorcluster)  [unwired: 8 in]
                    }
                    n181 = Merge Errors(w468) -> (w465:errorcluster)
                    n182 = case shown="No Error" w465 {
                      selector: w465 -> [w469 w470]
                      tunnel: [w469 w470] -> w462
                      frame No Error {
                      }
                      frame Error {
                      }
                    }
                  }
                }
                n183 = case shown="No Error" w438 {
                  tunnel: [Station_Action."Wait Item In" Station_Action."ImformOut"] -> w437
                  frame No Error {
                  }
                  frame Error {
                  }
                }
              }
              frame 3 {
                w498 = T8[] [enum."S3 動作完成_39"] items=["S2站PC動作中_20", "電流量測完成產品OK_21", "電流量測完成產品NG_22", "S2站Format 執行_23", "S2 Format OK_24", "S2 Format NG_25", "S2站燒入執行_26", "S2站燒入OK_27", "S2站燒入NG_28", "S2站動作完成_29", "S3 PC動作中_30", "S3 Format 此站執行_31", "S3 Format OK_32", "S3 Format NG_33", "S3 燒入程式 此站執行_34", "S3 燒入程式 OK_35", "S3 燒入程式 NG_36", "S3 備用_37", "S3 備用_38", "S3 動作完成_39", "S4 PC動作中_40", "S4 量測完成 產品正常_41", "S4 量測完成 產品NG_42", "S4 Format 此站執行_43", "S4 Format OK_44", "S4 Format NG_45", "S4 燒入 此站不執行_46", "S4 燒入程式 OK_47", "S4 燒入程式 NG_48", "S4 藍芽Scan OK_49", "S4 藍芽Scan NG_50", "S4 動作完成_51", "給PLC要量電流訊號", "給PLC要量電壓訊號"]
                n184 = Add(x=w498, y=20) -> (x+y=w506:i32[])
                n185 = for {
                  tunnel: [w512] -> w505 mode=indexing
                  tunnel: w500 -> [w511]
                  tunnel: w506 -> [w510] mode=indexing
                  tunnel: bool[] [TRUE] ("Sat Coils") -> [w509]
                  n186 = Wait (ms)(milliseconds to wait=100) -> ()  [unwired: 1 out]
                  n187 = Bundle(cluster=T4 {"starting address"=0, "number of inputs"=0, "Sat Coils"=[], "Holding Registers"=[]} ("data"), "starting address"=w510, "number of inputs"=u16 0, "Sat Coils"=w509) -> (w515:T4)  [unwired: 1 in]
                  n188 = call "ModbusCmdIn.vi"("error in (no error)"=w511, "data"=w515, "Enum"=ModbusCmd."Set Coils") -> ("error out"=w512:errorcluster)  [unwired: 8 in]
                }
                n189 = Merge Errors(w505) -> (w504:errorcluster)
                n190 = while {
                  tunnel: w497 -> [w548]
                  tunnel: w496 -> [w547]
                  tunnel: [w540] -> w503
                  tunnel: [w543] -> w502
                  tunnel: w504 -> [w537]
                  stop <- w544 stop-if-true
                  n191 = property class="Bool (strict)"(reference=w547) -> ("Value"=w546:bool)  [unwired: 1 in, 2 out]
                  n192 = Not(x=w546) -> (.not. x?=w545:bool)
                  n193 = call "INWait_Name.vi"("FlowCtrl in"=w548, "Input2"=Auto_Inspection_IN_Name2."S3 Tool Prpgram", "Wait?"=FALSE, "error in (no error)"=w537) -> ("StatusOut"=w542:bool, "error out"=w543:errorcluster)  [unwired: 8 in, 2 out]
                  n194 = Equal?(x=FALSE, y=w542) -> (x = y?=w540:bool)
                  n195 = Compound Arithmetic op=OR(w537, w540, w545) -> (w544:bool)
                  n196 = Wait (ms)(milliseconds to wait=123) -> ()  [unwired: 1 out]
                }
                n197 = case shown="True" w503 {
                  tunnel: w502 -> [w518 w524]
                  tunnel: [w518 w521] -> w493
                  tunnel: w495 -> [_ _]
                  frame False {
                  }
                  frame True {
                    w519 = T8[] [enum."S3 PC動作中_30", enum."S3 Format OK_32", enum."S3 Format NG_33", enum."S3 燒入程式 OK_35", enum."S3 燒入程式 NG_36", enum."S3 動作完成_39"] items=["S2站PC動作中_20", "電流量測完成產品OK_21", "電流量測完成產品NG_22", "S2站Format 執行_23", "S2 Format OK_24", "S2 Format NG_25", "S2站燒入執行_26", "S2站燒入OK_27", "S2站燒入NG_28", "S2站動作完成_29", "S3 PC動作中_30", "S3 Format 此站執行_31", "S3 Format OK_32", "S3 Format NG_33", "S3 燒入程式 此站執行_34", "S3 燒入程式 OK_35", "S3 燒入程式 NG_36", "S3 備用_37", "S3 備用_38", "S3 動作完成_39", "S4 PC動作中_40", "S4 量測完成 產品正常_41", "S4 量測完成 產品NG_42", "S4 Format 此站執行_43", "S4 Format OK_44", "S4 Format NG_45", "S4 燒入 此站不執行_46", "S4 燒入程式 OK_47", "S4 燒入程式 NG_48", "S4 藍芽Scan OK_49", "S4 藍芽Scan NG_50", "S4 動作完成_51", "給PLC要量電流訊號", "給PLC要量電壓訊號"]
                    n198 = Add(x=w519, y=20) -> (x+y=w523:i32[])
                    n199 = for {
                      tunnel: w523 -> [w528] mode=indexing
                      tunnel: [w530] -> w525 mode=indexing
                      tunnel: w524 -> [w529]
                      n200 = Wait (ms)(milliseconds to wait=100) -> ()  [unwired: 1 out]
                      n201 = Bundle(cluster=T4 {"starting address"=0, "number of inputs"=0, "Sat Coils"=[], "Holding Registers"=[]} ("data"), "starting address"=w528, "number of inputs"=u16 0, "Sat Coils"=bool[] [FALSE]) -> (w533:T4)  [unwired: 1 in]
                      n202 = call "ModbusCmdIn.vi"("error in (no error)"=w529, "data"=w533, "Enum"=ModbusCmd."Set Coils") -> ("error out"=w530:errorcluster)  [unwired: 8 in]
                    }
                    n203 = Merge Errors(w525) -> (w522:errorcluster)
                    n204 = case shown="Error .." w522 {
                      selector: w522 -> [w526 w527]
                      tunnel: [w526 w527] -> w521
                      frame No Error {
                      }
                      frame Error {
                      }
                    }
                  }
                }
                n205 = case shown="No Error" w493 {
                  tunnel: [Station_Action."Wait Item In" Station_Action."ImformOut"] -> w494
                  frame No Error {
                  }
                  frame Error {
                  }
                }
              }
              frame 4 {
                w550 = T8[] [enum."S4 動作完成_51"] items=["S2站PC動作中_20", "電流量測完成產品OK_21", "電流量測完成產品NG_22", "S2站Format 執行_23", "S2 Format OK_24", "S2 Format NG_25", "S2站燒入執行_26", "S2站燒入OK_27", "S2站燒入NG_28", "S2站動作完成_29", "S3 PC動作中_30", "S3 Format 此站執行_31", "S3 Format OK_32", "S3 Format NG_33", "S3 燒入程式 此站執行_34", "S3 燒入程式 OK_35", "S3 燒入程式 NG_36", "S3 備用_37", "S3 備用_38", "S3 動作完成_39", "S4 PC動作中_40", "S4 量測完成 產品正常_41", "S4 量測完成 產品NG_42", "S4 Format 此站執行_43", "S4 Format OK_44", "S4 Format NG_45", "S4 燒入 此站不執行_46", "S4 燒入程式 OK_47", "S4 燒入程式 NG_48", "S4 藍芽Scan OK_49", "S4 藍芽Scan NG_50", "S4 動作完成_51", "給PLC要量電流訊號", "給PLC要量電壓訊號"]
                n206 = Add(x=w550, y=20) -> (x+y=w562:i32[])
                n207 = for {
                  tunnel: [w568] -> w561 mode=indexing
                  tunnel: w554 -> [w567]
                  tunnel: w562 -> [w566] mode=indexing
                  tunnel: bool[] [TRUE] ("Sat Coils") -> [w565]
                  n208 = Wait (ms)(milliseconds to wait=100) -> ()  [unwired: 1 out]
                  n209 = Bundle(cluster=T4 {"starting address"=0, "number of inputs"=0, "Sat Coils"=[], "Holding Registers"=[]} ("data"), "starting address"=w566, "number of inputs"=u16 0, "Sat Coils"=w565) -> (w571:T4)  [unwired: 1 in]
                  n210 = call "ModbusCmdIn.vi"("error in (no error)"=w567, "data"=w571, "Enum"=ModbusCmd."Set Coils") -> ("error out"=w568:errorcluster)  [unwired: 8 in]
                }
                n211 = Merge Errors(w561) -> (w560:errorcluster)
                n212 = while {
                  tunnel: w553 -> [w616]
                  tunnel: w552 -> [w615]
                  tunnel: [w608] -> w559
                  tunnel: [w611] -> w558
                  tunnel: w560 -> [w605]
                  stop <- w612 stop-if-true
                  n213 = property class="Bool (strict)"(reference=w615) -> ("Value"=w614:bool)  [unwired: 1 in, 2 out]
                  n214 = Not(x=w614) -> (.not. x?=w613:bool)
                  n215 = call "INWait_Name.vi"("FlowCtrl in"=w616, "Input2"=Auto_Inspection_IN_Name2."S4 Tool Sacn", "Wait?"=FALSE, "error in (no error)"=w605) -> ("StatusOut"=w610:bool, "error out"=w611:errorcluster)  [unwired: 8 in, 2 out]
                  n216 = Equal?(x=FALSE, y=w610) -> (x = y?=w608:bool)
                  n217 = Compound Arithmetic op=OR(w605, w608, w613) -> (w612:bool)
                  n218 = Wait (ms)(milliseconds to wait=123) -> ()  [unwired: 1 out]
                }
                n219 = case shown="True" w559 {
                  tunnel: w558 -> [w574 w580]
                  tunnel: [w574 w577] -> w556
                  frame False {
                  }
                  frame True {
                    w575 = T8[] [enum."S4 PC動作中_40", enum."S4 量測完成 產品正常_41", enum."S4 量測完成 產品NG_42", enum."S4 Format OK_44", enum."S4 Format NG_45", enum."S4 燒入程式 OK_47", enum."S4 燒入程式 NG_48", enum."S4 藍芽Scan OK_49", enum."S4 藍芽Scan NG_50", enum."S4 動作完成_51", enum."給PLC要量電壓訊號"] items=["S2站PC動作中_20", "電流量測完成產品OK_21", "電流量測完成產品NG_22", "S2站Format 執行_23", "S2 Format OK_24", "S2 Format NG_25", "S2站燒入執行_26", "S2站燒入OK_27", "S2站燒入NG_28", "S2站動作完成_29", "S3 PC動作中_30", "S3 Format 此站執行_31", "S3 Format OK_32", "S3 Format NG_33", "S3 燒入程式 此站執行_34", "S3 燒入程式 OK_35", "S3 燒入程式 NG_36", "S3 備用_37", "S3 備用_38", "S3 動作完成_39", "S4 PC動作中_40", "S4 量測完成 產品正常_41", "S4 量測完成 產品NG_42", "S4 Format 此站執行_43", "S4 Format OK_44", "S4 Format NG_45", "S4 燒入 此站不執行_46", "S4 燒入程式 OK_47", "S4 燒入程式 NG_48", "S4 藍芽Scan OK_49", "S4 藍芽Scan NG_50", "S4 動作完成_51", "給PLC要量電流訊號", "給PLC要量電壓訊號"]
                    n220 = Add(x=w575, y=20) -> (x+y=w579:i32[])
                    n221 = for {
                      tunnel: w579 -> [w596] mode=indexing
                      tunnel: [w598] -> w581 mode=indexing
                      tunnel: w580 -> [w597]
                      n222 = Wait (ms)(milliseconds to wait=100) -> ()  [unwired: 1 out]
                      n223 = Bundle(cluster=T4 {"starting address"=0, "number of inputs"=0, "Sat Coils"=[], "Holding Registers"=[]} ("data"), "starting address"=w596, "number of inputs"=u16 0, "Sat Coils"=bool[] [FALSE]) -> (w601:T4)  [unwired: 1 in]
                      n224 = call "ModbusCmdIn.vi"("error in (no error)"=w597, "data"=w601, "Enum"=ModbusCmd."Set Coils") -> ("error out"=w598:errorcluster)  [unwired: 8 in]
                    }
                    n225 = Merge Errors(w581) -> (w578:errorcluster)
                    n226 = case shown="No Error" w578 {
                      selector: w578 -> [w582 w595]
                      tunnel: [w583 w595] -> w577
                      frame No Error {
                        n227 = disable-structure shown="Disabled" {
                          disable-tunnel: [w592 _] -> w583
                          disable-tunnel: w582 -> [w591 _]
                          frame Disabled {
                            # "收尋S4站條碼"
                            n228 = global read "Main Glb.vi" "Input Registers0-99"() -> (w590:u16[])
                            n229 = call "Red PLC InReg.vi"("length"=10, "index"=40, "Input Registers Arr"=w590) -> ("Rad In Reg"=w589:string)  [unwired: 7 in, 1 out]
                            n230 = call "Table Sav and Del.vi"("error in (no error)"=w591, "SN"=w589) -> ("error out"=w585:errorcluster, "未找到條碼"=w586:bool)  [unwired: 8 in]
                            n231 = case shown="True" w586 {
                              tunnel: [_ w593] -> w584
                              frame False {
                              }
                              frame True {
                                n232 = disable-structure shown="Disabled" {
                                disable-tunnel: [errorcluster {"status"=TRUE, "code"=18407, "source"=""} ("error in (no error)") _] -> w593
                                frame Disabled {
                                }
                                frame Enabled {
                                }
                                }
                              }
                            }
                            n233 = Merge Errors(w585, w584) -> (w592:errorcluster)
                          }
                          frame Enabled {
                          }
                        }
                      }
                      frame Error {
                      }
                    }
                  }
                }
                n234 = case shown="No Error" w556 {
                  tunnel: [Station_Action."Wait Item In" Station_Action."ImformOut"] -> w555
                  frame No Error {
                  }
                  frame Error {
                  }
                }
              }
              frame 5 {
                w618 = T9[] [enum."S11雷射測高完成"] items=["S11雷射測量動作中", "S11雷射測點1完成", "S11雷射測點2完成", "S11雷測測量OK", "S11雷測測量NG", "S11雷測測量重測", "S11備用_6", "S11備用_7", "S11備用_8", "S11雷射測高完成"]
                n235 = Add(x=w618, y=110) -> (x+y=w630:i32[])
                n236 = for {
                  tunnel: [w636] -> w629 mode=indexing
                  tunnel: w624 -> [w635]
                  tunnel: w630 -> [w634] mode=indexing
                  tunnel: bool[] [TRUE] ("Sat Coils") -> [w633]
                  n237 = Wait (ms)(milliseconds to wait=100) -> ()  [unwired: 1 out]
                  n238 = Bundle(cluster=T4 {"starting address"=0, "number of inputs"=0, "Sat Coils"=[], "Holding Registers"=[]} ("data"), "starting address"=w634, "number of inputs"=u16 0, "Sat Coils"=w633) -> (w639:T4)  [unwired: 1 in]
                  n239 = call "ModbusCmdIn.vi"("error in (no error)"=w635, "data"=w639, "Enum"=ModbusCmd."Set Coils") -> ("error out"=w636:errorcluster)  [unwired: 8 in]
                }
                n240 = Merge Errors(w629) -> (w628:errorcluster)
                n241 = while {
                  tunnel: w623 -> [w672]
                  tunnel: w622 -> [w671]
                  tunnel: [w664] -> w627
                  tunnel: [w667] -> w626
                  tunnel: w628 -> [w661]
                  stop <- w668 stop-if-true
                  n242 = property class="Bool (strict)"(reference=w671) -> ("Value"=w670:bool)  [unwired: 1 in, 2 out]
                  n243 = Not(x=w670) -> (.not. x?=w669:bool)
                  n244 = call "INWait_Name.vi"("FlowCtrl in"=w672, "Input2"=Auto_Inspection_IN_Name2."S11 Laser Detect", "Wait?"=FALSE, "error in (no error)"=w661) -> ("StatusOut"=w666:bool, "error out"=w667:errorcluster)  [unwired: 8 in, 2 out]
                  n245 = Equal?(x=FALSE, y=w666) -> (x = y?=w664:bool)
                  n246 = Compound Arithmetic op=OR(w661, w664, w669) -> (w668:bool)
                  n247 = Wait (ms)(milliseconds to wait=123) -> ()  [unwired: 1 out]
                }
                n248 = case shown="True" w627 {
                  tunnel: w626 -> [w642 w648]
                  tunnel: [w642 w645] -> w620
                  frame False {
                  }
                  frame True {
                    w643 = T9[] [enum."S11雷射測量動作中", enum."S11雷射測點1完成", enum."S11雷射測點2完成", enum."S11雷測測量OK", enum."S11雷測測量NG", enum."S11雷測測量重測", enum."S11雷射測高完成"] items=["S11雷射測量動作中", "S11雷射測點1完成", "S11雷射測點2完成", "S11雷測測量OK", "S11雷測測量NG", "S11雷測測量重測", "S11備用_6", "S11備用_7", "S11備用_8", "S11雷射測高完成"]
                    n249 = Add(x=w643, y=110) -> (x+y=w647:i32[])
                    n250 = for {
                      tunnel: w647 -> [w652] mode=indexing
                      tunnel: [w654] -> w649 mode=indexing
                      tunnel: w648 -> [w653]
                      n251 = Wait (ms)(milliseconds to wait=100) -> ()  [unwired: 1 out]
                      n252 = Bundle(cluster=T4 {"starting address"=0, "number of inputs"=0, "Sat Coils"=[], "Holding Registers"=[]} ("data"), "starting address"=w652, "number of inputs"=u16 0, "Sat Coils"=bool[] [FALSE]) -> (w657:T4)  [unwired: 1 in]
                      n253 = call "ModbusCmdIn.vi"("error in (no error)"=w653, "data"=w657, "Enum"=ModbusCmd."Set Coils") -> ("error out"=w654:errorcluster)  [unwired: 8 in]
                    }
                    n254 = Merge Errors(w649) -> (w646:errorcluster)
                    n255 = case shown="No Error" w646 {
                      selector: w646 -> [w650 w651]
                      tunnel: [w650 w651] -> w645
                      frame No Error {
                      }
                      frame Error {
                      }
                    }
                  }
                }
                n256 = case shown="No Error" w620 {
                  tunnel: [Station_Action."Wait Item In" Station_Action."ImformOut"] -> w621
                  frame No Error {
                  }
                  frame Error {
                  }
                }
              }
            }
          }
        }
        n257 = Number To Decimal String(number=w36) -> (decimal integer string=w37:string)  [unwired: 1 in]
        n258 = call-dynamic "Write FGV Data.vi"("Station Action in"=w35, "0Cv/1St"=1, "DataIn"=w37) -> ("Station Action out"=w34:refnum<class "Station Action.lvclass">)  [unwired: 11 in, 1 out]
        n259 = case shown="Error .." w33 {
          selector: w33 -> [_ w72]
          tunnel: w34 -> [_ w71]
          frame No Error {
          }
          frame Error {
            w66 = Auto_Inspection_Data_Name."LocalRun" ("Data")
            w63 = "0" ("DataIn")
            n260 = call-dynamic "WriteFGVError.vi"("error in (no error)"=w72, "0Cv/1St"=1, "Station Action in"=w71) -> ("error out"=w64:errorcluster, "Station Action out"=w67:refnum<class "Station Action.lvclass">)  [unwired: 7 in]
            n261 = call-dynamic "Write FGV Data.vi"("Station Action in"=w67, "0Cv/1St"=0, "DataIn"=w63, "Data"=w66, "error in (no error)"=w64) -> ("Station Action out"=w68:refnum<class "Station Action.lvclass">, "error out"=w65:errorcluster)  [unwired: 9 in]
            n262 = call-dynamic "Write FGV Data.vi"("Station Action in"=w68, "0Cv/1St"=1, "DataIn"=w63, "Data"=w66, "error in (no error)"=w65) -> ("error out"=w62:errorcluster)  [unwired: 9 in, 1 out]
            n263 = call <vilib>:"Clear Errors.vi"("error in (no error)"=w62) -> ()  [unwired: 5 in, 2 out]
          }
        }
        n264 = case shown="Error .." w33 {
          frame No Error {
          }
          frame Error {
            # "PC Alarm"
            # "PC-->PLC  PC Auto"
            n265 = Bundle(cluster=T4 {"starting address"=0, "number of inputs"=0, "Sat Coils"=[], "Holding Registers"=[]} ("data"), "starting address"=6, "number of inputs"=u16 0, "Sat Coils"=bool[] [TRUE]) -> (w55:T4)  [unwired: 1 in]
            n266 = Bundle(cluster=T4 {"starting address"=0, "number of inputs"=0, "Sat Coils"=[], "Holding Registers"=[]} ("data"), "starting address"=1, "number of inputs"=u16 0, "Sat Coils"=bool[] [FALSE]) -> (w56:T4)  [unwired: 1 in]
            n267 = call "ModbusCmdIn.vi"("data"=w56, "Enum"=ModbusCmd."Set Coils") -> ("error out"=w49:errorcluster)  [unwired: 9 in]
            n268 = call "ModbusCmdIn.vi"("error in (no error)"=w49, "data"=w55, "Enum"=ModbusCmd."Set Coils") -> ("error out"=w48:errorcluster)  [unwired: 8 in]
            n269 = call <vilib>:"Clear Errors.vi"("error in (no error)"=w48) -> ()  [unwired: 5 in, 2 out]
          }
        }
        n270 = property class="Enum (strict)"(reference=w44, "Value"=w36) -> ()  [unwired: 1 in, 2 out]
      }
    }
    n271 = call "Exit.vi"() -> ("ExitOut"=w19:bool)  [unwired: 11 in]
  }
  n272 = disable-structure shown="Disabled" {
    frame Disabled {
      n273 = case shown="0, Default" {
        selector: _ -> [_ _ _ _ _ _]
        tunnel: [Auto_Inspection_IN_Name2."S0 Station" Auto_Inspection_IN_Name2."S1 Barcode " Auto_Inspection_IN_Name2."S2 Tool Format" Auto_Inspection_IN_Name2."S3 Tool Prpgram" Auto_Inspection_IN_Name2."S4 Tool Sacn" Auto_Inspection_IN_Name2."S11 Laser Detect"] -> w674
        frame 0, Default {
        }
        frame 1 {
        }
        frame 2 {
        }
        frame 3 {
        }
        frame 4 {
        }
        frame 5 {
        }
      }
      n274 = call "INWait_Name.vi"("Input2"=w674) -> ()  [unwired: 11 in, 4 out]
    }
    frame Enabled {
    }
  }
  n275 = disable-structure shown="Disabled" {
    disable-tunnel: _ -> [w681 _]
    frame Disabled {
      n276 = call "Auto Inspection_Status.vi"("Action"=enum16{"Initial", "Write", "Read"}."Write", "DataIn"="wait input", "Station"=Auto_Inspection_Station_Name2."S1Barcode", "Data"=Auto_Inspection_Data_Name."CurrentAction", "error in"=w681) -> ()  [unwired: 8 in, 3 out]
    }
    frame Enabled {
    }
  }
  n277 = disable-structure shown="Disabled" {
    frame Disabled {
      n278 = flat-sequence {
        tunnel: _ -> [w700]
        tunnel: _ -> [w698]
        frame #0 {
          n279 = Variant To Data(type=T11 {"LineScan arrive"=refnum, "LineScanfinish"=refnum, "AI arrive"=refnum, "AI finish"=refnum, "NG Pick arrive"=refnum, "NG Pick finish"=refnum} ("UI Ref"), Variant=w698) -> (data=w690:T11)  [unwired: 1 in, 1 out]
          n280 = call-dynamic "Read UIRef.vi"("0Arrive/1Finish"=1, "UI Ref"=w690, "Station Action in"=w700) -> ("error out"=w693:errorcluster, "RefOut"=w699:refnum<vi>, "Station Action out"=w694:refnum<class "Station Action.lvclass">)  [unwired: 6 in]
          n281 = property class="Bool (strict)"(reference=w699, error in=w693, "Value"=TRUE) -> (reference out=w687:refnum<vi>, error out=w692:errorcluster)
          n282 = call-dynamic "Read UIRef.vi"("error in (no error)"=w692, "0Arrive/1Finish"=0, "UI Ref"=w690, "Station Action in"=w694) -> ("RefOut"=w689:refnum<vi>)  [unwired: 5 in, 2 out]
          n283 = while {
            tunnel: w689 -> [w706]
            tunnel: [w701] -> w686
            stop <- w705 stop-if-true
            n284 = property on="Property Node" class="Bool (strict)"(reference=w706) -> (error out=w701:errorcluster, "Value"=w704:bool)  [unwired: 1 in, 1 out]
            n285 = Wait (ms)(milliseconds to wait=u32 33) -> ()  [unwired: 1 out]
            n286 = Equal?(x=w704, y=FALSE) -> (x = y?=w705:bool)
          }
          n287 = property class="Bool (strict)"(reference=w687, error in=w686, "Value"=FALSE) -> ()  [unwired: 2 out]
        }
      }
    }
    frame Enabled {
    }
  }
